vi "Test Customer Pick Up Last Order Item Stops if in App Context.vi"(8 "error in (no error)":errorcluster, 11 "Customer Test in":refnum<class "Customer Test.lvclass">=refnum) -> (0 "error out":errorcluster, 3 "Customer Test out":refnum<class "Customer Test.lvclass">)   [LabVIEW 2020, in "Customer Test.lvclass"]
uses:
  Customer Test.lvclass
  Processes/People/Customers/Customer/Customer.lvclass
  Support/Beverages/Beverage/Beverage.lvclass
  <vilib>/Astemes/Triarc Framework/Process/Process.lvclass
  Support/Beverages/TypeDefs/Options.ctl
  Support/Beverages/TypeDefs/Drink Type.ctl
  <vilib>/Astemes/Triarc Framework/Process/Public/Lifecycle/Lifecycle State.ctl
  <vilib>/Astemes/LUnit/Test Case.lvclass
  <vilib>/Astemes/Triarc Framework/Application/Application.lvclass
  C:/Program Files (x86)/National Instruments/LabVIEW 2020/vi.lib/Astemes/Triarc Framework/Process/Process.lvclass
  C:/Program Files (x86)/National Instruments/LabVIEW 2020/vi.lib/Astemes/Triarc Framework/Base/Base.lvclass
  C:/Program Files (x86)/National Instruments/LabVIEW 2020/vi.lib/Astemes/Triarc Framework/Error Handler Interface/Error Handler Interface.lvclass
  C:/Program Files (x86)/National Instruments/LabVIEW 2020/vi.lib/Astemes/Triarc Framework/Logging/Logging.lvclass
  C:/Program Files (x86)/National Instruments/LabVIEW 2020/vi.lib/Astemes/Triarc Framework/Application/Application.lvclass
  C:/Program Files (x86)/National Instruments/LabVIEW 2020/vi.lib/Astemes/Triarc Framework/Async Handler/Async Handler.lvclass
  C:/git/astemes-triarc-examples/source/Coffee Shop/Processes/People/Person/Person.lvclass
  C:/Program Files (x86)/National Instruments/LabVIEW 2020/vi.lib/Astemes/Triarc Framework/View/View.lvclass
  C:/git/astemes-triarc-examples/source/Coffee Shop/Processes/People/Customers/Customer/Customer.lvclass
  C:/git/astemes-triarc-examples/source/Coffee Shop/Processes/People/Process Job/Job Handler.lvclass
  Test Doubles/Stub Job Handler/Stub Job Handler.lvclass
  Processes/People/Person/Person.lvclass
  C:/Program Files (x86)/National Instruments/LabVIEW 2020/vi.lib/Astemes/LUnit/Test Case.lvclass
  C:/Program Files (x86)/National Instruments/LabVIEW 2020/vi.lib/Astemes/LUnit/LUnit Runnable.lvclass
  C:/git/astemes-triarc-examples/source/Coffee Shop/Tests/Test Doubles/Stub Job Handler/Stub Job Handler.lvclass
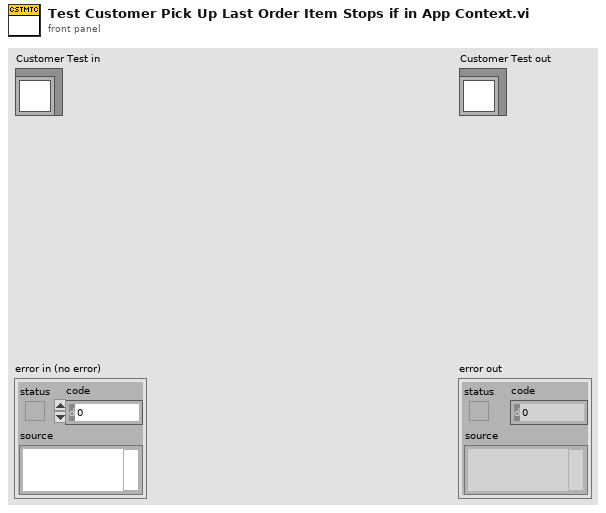
[diagram p1: front panel]
types:
  T1 = typedef "TF.lvlib/Process.lvclass/Lifecycle State.ctl" = enum16{"Uninitialized", "Initialized", "Started", "Running", "Stopped", "Finished"}
  T2 = typedef "Beverage.lvclass/Drink Type.ctl" = enum16{"Dark Roast", "Decaf", "Espresso", "House Blend"}
  T3 = typedef "Beverage.lvclass/Options.ctl" = enum16{"<None>", "Milk", "Mocha", "Soy", "Whip"}
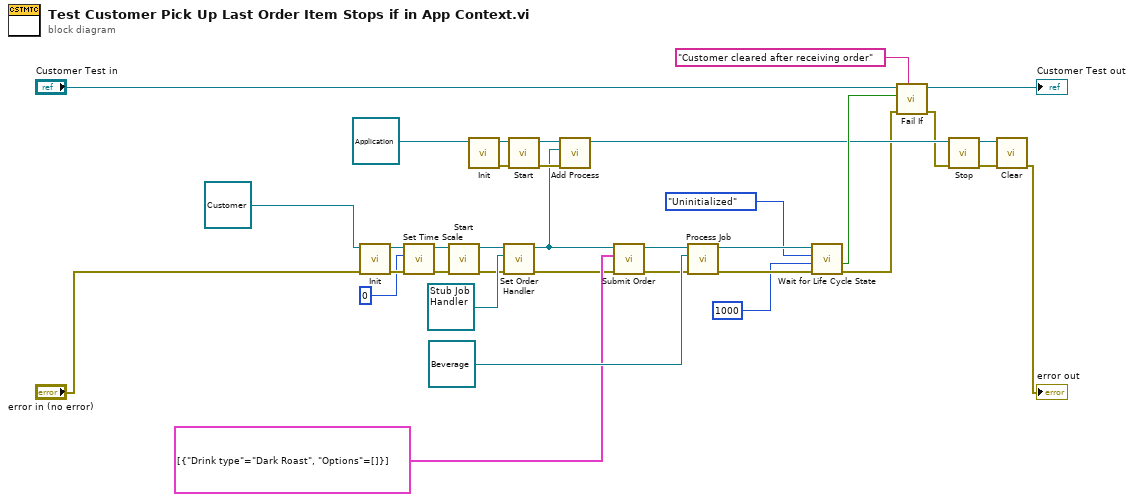
[diagram p0: block diagram]
diagram:
  n1 = call-dynamic "Init.vi"("error in (no error)"="error in (no error)", "View In"=refnum<class "Customer.lvclass"> refnum ("Customer.lvclass")) -> ("error out"=w34:errorcluster, "View Out"=w4:refnum<class "Customer.lvclass">)  [unwired: 8 in]
  n2 = call "Set Time Scale.vi"("TRIARC_ERROR_IN"=w34, "Time Scale [ms]"=u32 0, "Person In"=w4) -> ("TRIARC_ERROR_OUT"=w5:errorcluster, "Person Out"=w3:refnum<class "Customer.lvclass">)  [unwired: 7 in]
  n3 = call <vilib>:"Start.vi"("error in (no error)"=w5, "Process In"=w3) -> ("error out"=w8:errorcluster, "Process Out"=w7:refnum<class "Customer.lvclass">)  [unwired: 7 in, 1 out]
  n4 = call-dynamic "Init.vi"("Process In"=refnum<class "Application.lvclass"> refnum ("TF.lvlib:Application.lvclass")) -> ("error out"=w20:errorcluster, "Process Out"=w21:refnum<class "Application.lvclass">)  [unwired: 9 in]
  n5 = call "Set Order Handler.vi"("error in (no error)"=w8, "Order Handler"=refnum<class "Stub Job Handler.lvclass"> refnum ("Stub Job Handler.lvclass"), "Customer In"=w7) -> ("error out"=w11:errorcluster, "Customer Out"=w10:refnum<class "Customer.lvclass">)  [unwired: 7 in]
  n6 = call <vilib>:"Start.vi"("error in (no error)"=w20, "Process In"=w21) -> ("error out"=w17:errorcluster, "Process Out"=w18:refnum<class "Application.lvclass">)  [unwired: 7 in, 1 out]
  n7 = call <vilib>:"Add Process.vi"("error in (no error)"=w17, "Process"=w10, "Application In"=w18) -> ("Application Out"=w16:refnum<class "Application.lvclass">)  [unwired: 7 in, 1 out]
  n8 = call "Submit Order.vi"("error in (no error)"=w11, "Order Content"=cluster{"Drink type":T2, "Options":T3[]}[] [{"Drink type"=enum."Dark Roast", "Options"=[]}], "Customer In"=w10) -> ("error out"=w27:errorcluster, "Customer Out"=w26:refnum<class "Customer.lvclass">)  [unwired: 7 in]
  n9 = call-dynamic "Process Job.vi"("error in (no error)"=w27, "Job"=refnum<class "Beverage.lvclass"> refnum ("Beverage.lvclass"), "Process Job In"=w26) -> ("error out"=w33:errorcluster, "Process Job Out"=w28:refnum<class "Customer.lvclass">)  [unwired: 7 in]
  n10 = call <vilib>:"Wait for Life Cycle State.vi"("error in (no error)"=w33, "timeout in ms (-1)"=1000, "Lifecycle State"=Lifecycle_State."Uninitialized", "Process In"=w28) -> ("error out"=w6:errorcluster, "timed out?"=w22:bool)  [unwired: 5 in, 1 out]
  n11 = call <vilib>:"Fail If.vi"("Description"="Customer cleared after receiving order", "error in (no error)"=w6, "Fail?"=w22, "LUnit Test Case In"="Customer Test in") -> ("error out"=w13:errorcluster, "LUnit Test Case Out"=→"Customer Test out":refnum<class "Test Case.lvclass">)  [unwired: 6 in]
  n12 = call <vilib>:"Stop.vi"("error in (no error)"=w13, "Process In"=w16) -> ("error out"=w14:errorcluster, "Process Out"=w15:refnum<class "Application.lvclass">)  [unwired: 7 in, 1 out]
  n13 = call-dynamic "Clear.vi"("error in (no error)"=w14, "Application In"=w15) -> ("error out"=→"error out":errorcluster)  [unwired: 9 in]
